vi "LDA_Autocorrelation2.vi"(0 "U":dbl[](array[numeric]) format="%.2f", 2 "Total times":dbl[](array[numeric]) format="%.2f") -> (3 "Delta T":dbl format="%.2f")   [LabVIEW 2010]
panel:
  out "No of points":i32[](graph)
  out "Auto-Corr":cluster{dbl, "Delta T":dbl, dbl[]}(graph)
  out "No of points":i32[](array[numeric])
  out "Products":dbl[](array[numeric]) format="%.2f"
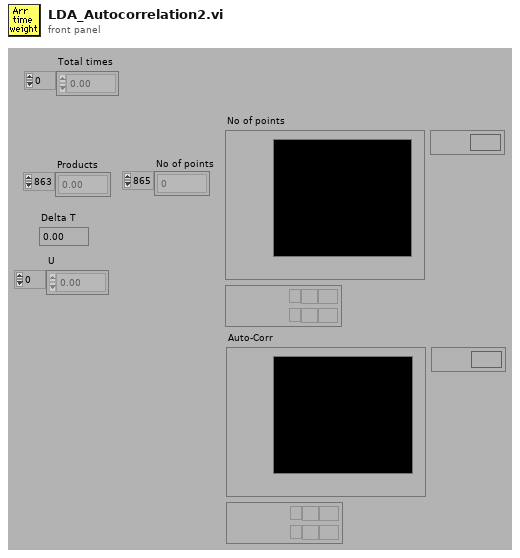
[diagram p1: front panel]
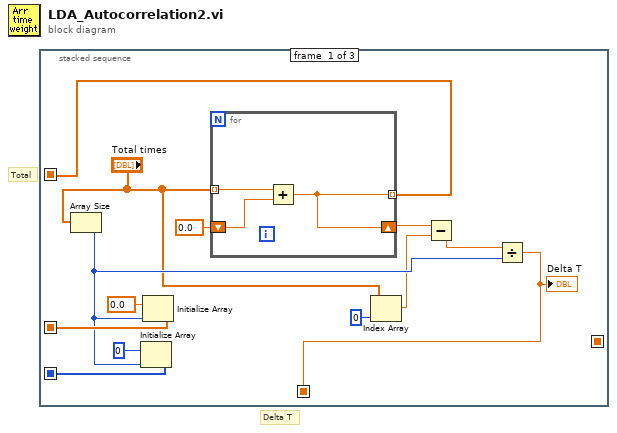
[diagram p0: block diagram]
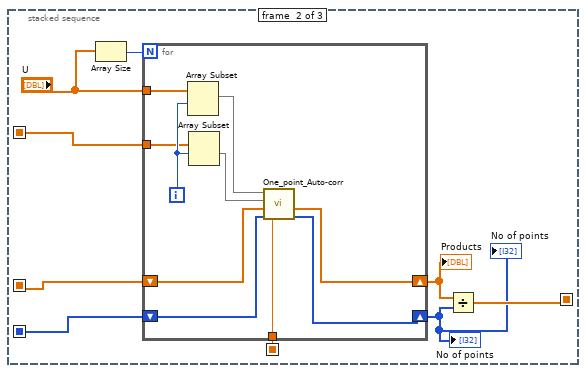
[diagram p2: hidden frame]
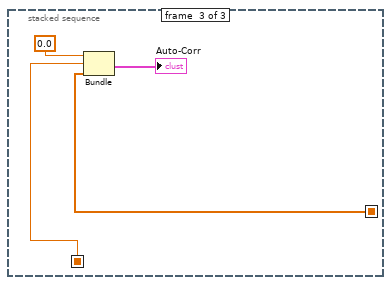
[diagram p3: hidden frame]
diagram:
  # "Delta T"
  # "Total"
  n1 = stacked-sequence {
    seq-local: [w12 _ _] -> [_ w23 _]
    seq-local: [w9 _ _] -> [_ w25 _]
    seq-local: [w8 _ _] -> [_ w24 _]
    seq-local: [_ w20 _] -> [_ _ w39]
    seq-local: [w6 _ _] -> [_ w17 w37]
    frame #0 {
      n2 = Array Size(array="Total times") -> (size(s)=w7:i32)
      n3 = Initialize Array(0, w7) -> (w9:i32[])
      n4 = Initialize Array(0.0, w7) -> (w8:dbl[])
      n5 = for {
        shift-right: [w14] -> w3
        shift-left: 0.0 -> [w15]
        tunnel: "Total times" -> [w16] mode=indexing
        tunnel: [w14] -> w12 mode=indexing
        n6 = Add(x=w16, y=w15) -> (x+y=w14:dbl)
      }
      n7 = Index Array(array="Total times", index=0) -> (element=w2:dbl)
      n8 = Subtract(x=w3, y=w2) -> (x-y=w1:dbl)
      n9 = Divide(x=w1, y=w7) -> (x/y=w6:dbl)
      "Delta T" <- w6
    }
    frame #1 {
      n10 = Array Size(array="U") -> (size(s)=w22:i32)
      n11 = for {
        N: w22 -> [_]
        shift-right: [w28] -> w21
        shift-left: w24 -> [w34]
        shift-right: [w27] -> w19
        shift-left: w25 -> [w35]
        tunnel: w23 -> [w32]
        tunnel: "U" -> [w29]
        tunnel: w17 -> [w26]
        i -> [w33]
        n12 = Array Subset(array=w29, index=w33) -> (w30:dbl[])  [unwired: 1 in]
        n13 = Array Subset(array=w32, index=w33) -> (w31:dbl[])  [unwired: 1 in]
        n14 = call "One_point_Auto-corr.vi"("Delta T"=w26, "No of products in"=w35, "Auto-corr in"=w34, "Total Arr times"=w31, "U"=w30) -> ("No of products out"=w27:i32[], "Auto-corr out"=w28:dbl[])  [unwired: 4 in]
      }
      "Products" <- w21
      "No of points" <- w19
      "No of points" <- w19
      n15 = Divide(x=w21, y=w19) -> (x/y=w20:dbl[])
    }
    frame #2 {
      n16 = Bundle(0.0, w37, w39) -> (→"Auto-Corr":cluster{dbl, dbl, dbl[]})  [unwired: 1 in]
    }
  }
